vi "Merge CfgTables.vi"(7 "Reference CfgTable":string[][](array[string]), 8 "error in (no error)":errorcluster, 10 "Key Index":i32, 11 "CfgTable Row in":string[][](array[string])) -> (0 "error out":errorcluster, 3 "CfgTable Row out":string[][](array[string]))   [LabVIEW 2017, in "ClusterCfgTable.lvlib"]
doc: "Merges the rows of CfgTable Row in into Reference CfgTable, matching rows on the column given by Key Index. Rows whose key is not present are appended."
uses:
  ClusterCfgTable.lvlib
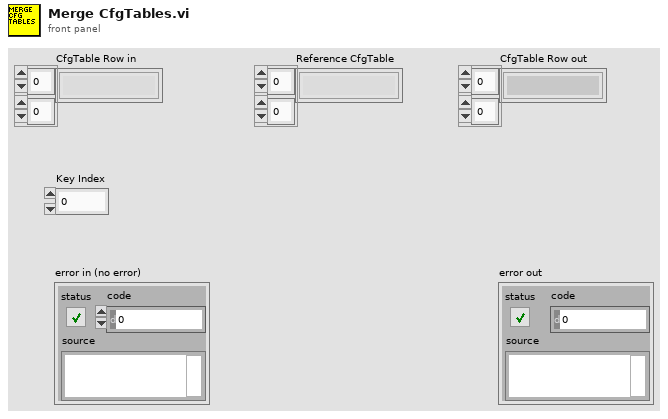
[diagram p1: front panel]
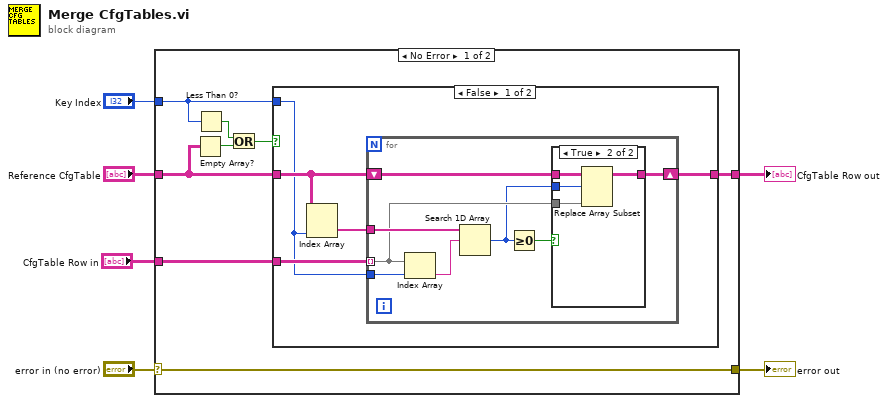
[diagram p0: block diagram]
diagram:
  n1 = case shown="No Error" "error in (no error)" {
    selector: "error in (no error)" -> [w12 w35]
    tunnel: "CfgTable Row in" -> [w14 w34]
    tunnel: [w13 w34] -> w2
    tunnel: "Key Index" -> [w8 _]
    tunnel: "Reference CfgTable" -> [w11 _]
    tunnel: [w12 w35] -> w6
    frame No Error {
      n2 = Empty Array?(array=w11) -> (empty?=w10:bool)
      n3 = Less Than 0?(x=w8) -> (x < 0?=w9:bool)
      n4 = Or(x=w9, y=w10) -> (x .or. y?=w7:bool)
      n5 = case shown="False" w7 {
        tunnel: w14 -> [w18 w33]
        tunnel: [w17 w33] -> w13
        tunnel: w11 -> [w16 _]
        tunnel: w8 -> [w15 _]
        frame False {
          n6 = Index Array(array=w16, index (col)=w15) -> (element=w19:string[])  [unwired: 1 in]
          n7 = for {
            shift-right: [w25] -> w17
            shift-left: w16 -> [w27]
            tunnel: w18 -> [w23] mode=indexing
            tunnel: w19 -> [w24]
            tunnel: w15 -> [w26]
            n8 = Index Array(array=w23, index=w26) -> (element=w22:string)
            n9 = Search 1D Array(1D array=w24, element=w22) -> (index of element=w21:i32)  [unwired: 1 in]
            n10 = Greater Or Equal To 0?(x=w21) -> (x >= 0?=w20:bool)
            n11 = case shown="True" w20 {
              tunnel: w27 -> [w28 w32]
              tunnel: [w28 w31] -> w25
              tunnel: w23 -> [_ w30]
              tunnel: w21 -> [_ w29]
              frame False {
              }
              frame True {
                n12 = Replace Array Subset(array=w32, new element=w30, index (row)=w29) -> (w31:string[][])  [unwired: 1 in]
              }
            }
          }
        }
        frame True {
        }
      }
    }
    frame Error {
    }
  }
  "error out" <- w6
  "CfgTable Row out" <- w2
